vi "Ctor.vi"(8 "error in (no error)":errorcluster, 11 "ByRef Mul in":refnum<class "ByRef Mul.lvclass">) -> (0 "error out":errorcluster, 3 "ByRef Mul out":refnum<class "ByRef Mul.lvclass">)   [LabVIEW 2020, in "ByRef Mul.lvclass"]
uses:
  ByRef Mul.lvclass
  ByRef Base/ByRef Base.lvclass
  Ref Data.ctl
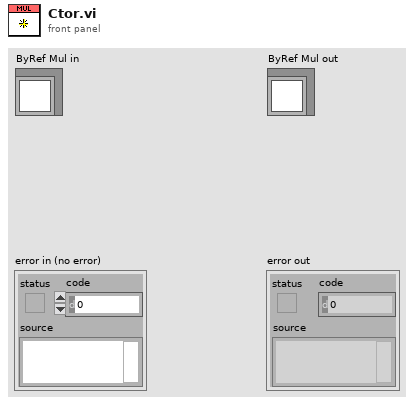
[diagram p1: front panel]
types:
  T1 = typedef "ByRef Mul.lvclass/Ref Data.ctl" = cluster{"To Mul":dbl}
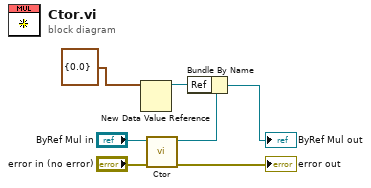
[diagram p0: block diagram]
diagram:
  n1 = New Data Value Reference(data value=T1 {"To Mul"=0.0} ("Ref Data")) -> (data value reference=w2:refnum<data-value>)  [unwired: 1 in, 1 out]
  n2 = call-parent "Ctor.vi"("error in (no error)"="error in (no error)", "ByRef Base in"="ByRef Mul in") -> ("error out"=→"error out":errorcluster, "ByRef Base out"=w3:refnum<class "ByRef Mul.lvclass">)  [unwired: 8 in]
  n3 = Bundle By Name(cluster=w3, "Ref"=w2) -> (→"ByRef Mul out":refnum<class "ByRef Mul.lvclass">)
